vi "VI Server_Get Picture Ring Selection.vi"(7 "Label":string, 8 "error in":errorcluster, 9 "Single Instance (T)":bool=TRUE, 11 "VI Server Cluster":T1) -> (0 "error out":errorcluster, 1 "Control Reference":refnum<vi>, 2 "Selection":string, 3 "VI Server Cluster.DUP":T1, 4 "Value":u16, 6 "Label.Text DUP":string)   [LabVIEW 2020, in "VI Server Toolkit LV2013.lvlib"]
doc: "Returns Item Name (picture) selected of the Picture Ring."
uses:
  VI Server Toolkit LV2013.lvlib
  VI Server_TypeDefs/VI Server_RefsCluster.ctl
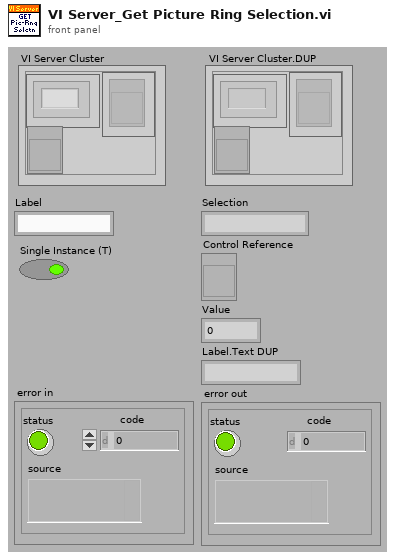
[diagram p1: front panel]
types:
  T1 = typedef "VI Server_RefsCluster.ctl" = cluster{"Labels":string[], "Refs":refnum<vi>[], "VI Ref":refnum<vi>}
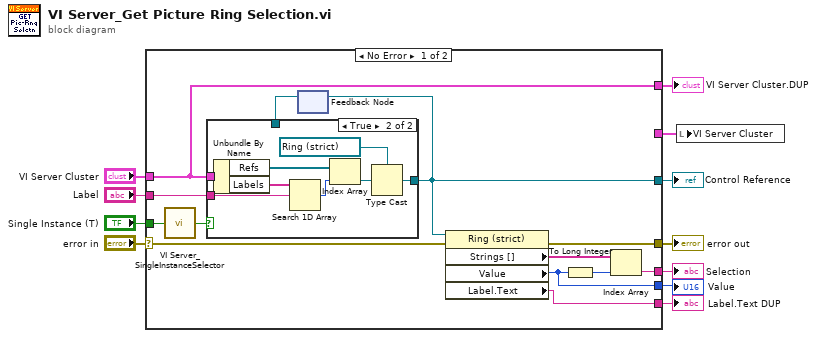
[diagram p0: block diagram]
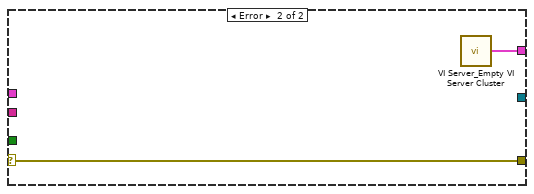
[diagram p3: hidden frame]
diagram:
  n1 = case shown="No Error" "error in" {
    selector: "error in" -> [w23 w35]
    tunnel: "Label" -> [w24 _]
    tunnel: "VI Server Cluster" -> [w12 _]
    tunnel: [w22 w35] -> w11
    tunnel: [w14 _] -> w7
    tunnel: [w19 _] -> w6
    tunnel: [w18 _] -> w5
    tunnel: [w17 _] -> w4
    tunnel: "Single Instance (T)" -> [w15 _]
    tunnel: [w12 _] -> w2
    tunnel: [_ w34] -> w1
    frame No Error {
      n2 = call "VI Server_SingleInstanceSelector.vi"("Single Instance (T)"=w15) -> ("Single Instance.OUT"=w16:bool)  [unwired: 6 in]
      n3 = feedback #1() -> (w13:refnum<vi>)  [unwired: 1 in]
      n4 = case shown="True" w16 {
        tunnel: w24 -> [_ w32]
        tunnel: w12 -> [_ w30]
        tunnel: [w25 w27] -> w14
        tunnel: w13 -> [w25 _]
        frame False {
        }
        frame True {
          n5 = Unbundle By Name(w30) -> ("Refs"=w29:refnum<vi>[], "Labels"=w33:string[])
          n6 = Search 1D Array(1D array=w33, element=w32) -> (index of element=w31:i32)  [unwired: 1 out]
          n7 = Index Array(array=w29, index=w31) -> (element=w28:refnum<vi>)
          n8 = Type Cast(type=refnum<vi> refnum ("Ring"), x=w28) -> (*(type *) &x=w27:refnum<vi>)
        }
      }
      n9 = feedback-in #1(w14) -> ()
      n10 = property class="Ring (strict)"(reference=w14, error in=w23) -> (error out=w22:errorcluster, "Strings []"=w21:string[], "Value"=w18:u16, "Label.Text"=w17:string)  [unwired: 1 out]
      n11 = To Long Integer(number=w18) -> (32bit integer=w20:i32)
      n12 = Index Array(array=w21, index=w20) -> (element=w19:string)
    }
    frame Error {
      n13 = call "VI Server_Empty VI Server Cluster.vi"() -> ("VI Server Cluster"=w34:T1)  [unwired: 7 in]
    }
  }
  "error out" <- w11
  "VI Server Cluster.DUP" <- w2
  "Control Reference" <- w7
  "Selection" <- w6
  "Value" <- w5
  "Label.Text DUP" <- w4
  n14 = local write "VI Server Cluster"(w1) -> ()
